vi "FirstByte to ControlPacket.vi"(7 "MQTTVersion":refnum<class "MQTTVersion.lvclass">, 11 "Packet First Byte":u8 format="%08b") -> (3 "Packet Type":refnum<class "ControlPacket.lvclass">)   [LabVIEW 2013, in "MQTT_Control_Packets.lvlib" / "MQTTVersion.lvclass"]
uses:
  MQTTVersion.lvclass
  ControlPacket/ControlPacket.lvclass
  CONNECT/CONNECT.lvclass
  CONNACK/CONNACK.lvclass
  PUBLISH/PUBLISH.lvclass
  PUBACK/PUBACK.lvclass
  PUBREC/PUBREC.lvclass
  PUBREL/PUBREL.lvclass
  PUBCOMP/PUBCOMP.lvclass
  SUBSCRIBE/SUBSCRIBE.lvclass
  SUBACK/SUBACK.lvclass
  UNSUBSCRIBE/UNSUBSCRIBE.lvclass
  UNSUBACK/UNSUBACK.lvclass
  PINGREQ/PINGREQ.lvclass
  PINGRESP/PINGRESP.lvclass
  DISCONNECT/DISCONNECT.lvclass
  ControlPacket/ControlPacket.lvclass/ControlPacket.ctl
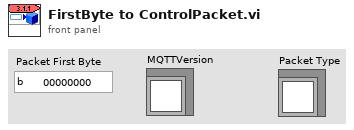
[diagram p1: front panel]
types:
  T1 = typedef "MQTT_Control_Packets.lvlib/ControlPacket.lvclass/Control Packet Type -- enum.ctl" = enum16{"Reserved", "CONNECT", "CONNACK", "PUBLISH", "PUBACK", "PUBREC", "PUBREL", "PUBCOMP", "SUBSCRIBE", "SUBACK", "UNSUBSCRIBE", "UNSUBACK", "PINGREQ", "PINGRESP", "DISCONNECT", "AUTH"}
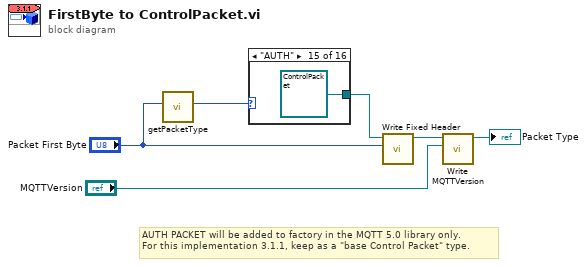
[diagram p0: block diagram]
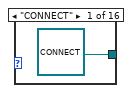
[diagram p2: hidden frame]
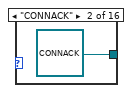
[diagram p3: hidden frame]
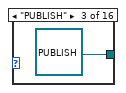
[diagram p4: hidden frame]
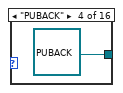
[diagram p5: hidden frame]
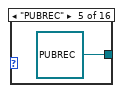
[diagram p6: hidden frame]
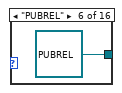
[diagram p7: hidden frame]
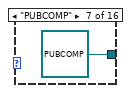
[diagram p8: hidden frame]
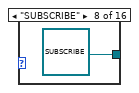
[diagram p9: hidden frame]
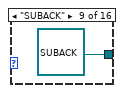
[diagram p10: hidden frame]
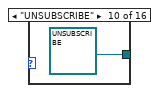
[diagram p11: hidden frame]
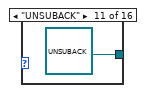
[diagram p12: hidden frame]
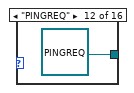
[diagram p13: hidden frame]
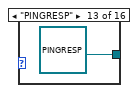
[diagram p14: hidden frame]
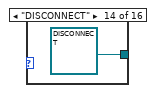
[diagram p15: hidden frame]
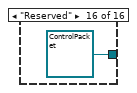
[diagram p16: hidden frame]
diagram:
  # "AUTH PACKET will be added to factory in the MQTT 5.0 library only.\nFor this implementation 3.1.1, keep as a \"base Control Packet\" type."
  n1 = call "getPacketType.vi"("Packet First Byte"="Packet First Byte") -> ("Control Packet Type"=w4:T1)  [unwired: 10 in]
  n2 = case shown="\"AUTH\"" w4 {
    tunnel: [refnum<class "CONNECT.lvclass"> refnum ("CONNECT.lvclass") refnum<class "CONNACK.lvclass"> refnum ("CONNACK.lvclass") refnum<class "PUBLISH.lvclass"> refnum ("PUBLISH.lvclass") refnum<class "PUBACK.lvclass"> refnum ("CONNECT.lvclass") refnum<class "PUBREC.lvclass"> refnum ("PUBREC.lvclass") refnum<class "PUBREL.lvclass"> refnum ("PUBREL.lvclass") refnum<class "PUBCOMP.lvclass"> refnum ("PUBCOMP.lvclass") refnum<class "SUBSCRIBE.lvclass"> refnum ("SUBSCRIBE.lvclass") refnum<class "SUBACK.lvclass"> refnum ("SUBACK.lvclass") refnum<class "UNSUBSCRIBE.lvclass"> refnum ("UNSUBSCRIBE.lvclass") refnum<class "UNSUBACK.lvclass"> refnum ("UNSUBACK.lvclass") refnum<class "PINGREQ.lvclass"> refnum ("PINGREC.lvclass") refnum<class "PINGRESP.lvclass"> refnum ("PINGRESP.lvclass") refnum<class "DISCONNECT.lvclass"> refnum ("DISCONNECT.lvclass") refnum<class "ControlPacket.lvclass"> refnum ("CONNACK.lvclass") refnum<class "ControlPacket.lvclass"> refnum ("CONNACK.lvclass")] -> w6
    frame "CONNECT" {
    }
    frame "CONNACK" {
    }
    frame "PUBLISH" {
    }
    frame "PUBACK" {
    }
    frame "PUBREC" {
    }
    frame "PUBREL" {
    }
    frame "PUBCOMP" {
    }
    frame "SUBSCRIBE" {
    }
    frame "SUBACK" {
    }
    frame "UNSUBSCRIBE" {
    }
    frame "UNSUBACK" {
    }
    frame "PINGREQ" {
    }
    frame "PINGRESP" {
    }
    frame "DISCONNECT" {
    }
    frame "AUTH" {
    }
    frame "Reserved" {
    }
  }
  n3 = call "Write Fixed Header.vi"("Fixed Header"="Packet First Byte", "ControlPacket in"=w6) -> ("ControlPacket out"=w3:refnum<class "ControlPacket.lvclass">)  [unwired: 9 in]
  n4 = call "Write MQTTVersion.vi"("MQTTVersion"="MQTTVersion", "ControlPacket in"=w3) -> ("ControlPacket out"=→"Packet Type":refnum<class "ControlPacket.lvclass">)  [unwired: 9 in]
